vi "Set Modbus.vi"(10 "Modbus":refnum<class "DesktopModbus.lvclass">, 11 "Model in":refnum<class "Model.lvclass">) -> (3 "Model out":refnum<class "Model.lvclass">)   [LabVIEW 2015, in "Model.lvclass"]
uses:
  Model.lvclass
  Modbus/DesktopModbus/DesktopModbus.lvclass
  Model.lvclass/Model.ctl
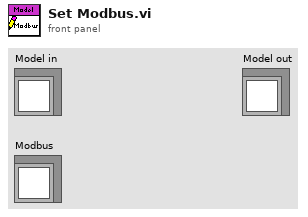
[diagram p1: front panel]
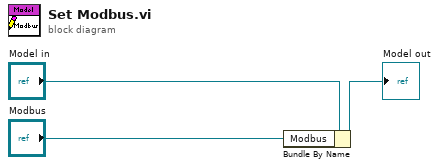
[diagram p0: block diagram]
diagram:
  n1 = Bundle By Name(cluster="Model in", "Modbus"="Modbus") -> (→"Model out":refnum<class "Model.lvclass">)
